vi "SOAE-Initialize Hardware.vi"(0 "Params":T1, 11 "error in (no error)":errorcluster) -> (4 "task out":refnum<k21>, 15 "error out":errorcluster)   [LabVIEW 2020]
uses:
  Typedefs/SOAE-Parameters.ctl
  Misc VIs/Connection Manager/Type Defs/Input sources.ctl
  <vilib>/DAQmx/create/channels.llb/DAQmx Create Channel (AI-Voltage-Basic).vi
  <vilib>/DAQmx/configure/timing.llb/DAQmx Timing (Sample Clock).vi
  <resource>/objmgr/daqmx.rc
panel:
  in  "input terminal configuration":i32(ring)=-1 items=["Default"=-1, "RSE"=10083, "NRSE"=10078, "Differential"=10106, "Pseudodifferential"=12529]
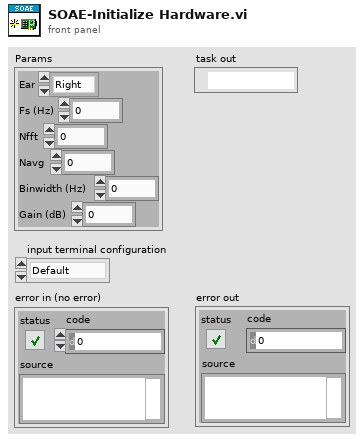
[diagram p1: front panel]
types:
  T1 = typedef "SOAE-Parameters.ctl" = cluster{"Ear":enum16{"Right", "Left"}, "Fs (Hz)":dbl, "Nfft":i32, "Navg":i32, "Binwidth (Hz)":dbl, "Gain (dB)":dbl}
  T2 = typedef "Input sources.ctl" = u16
  T3 = typedef "PXI-Device Spec.ctl" = cluster{"Slot":i32, "ProductType":string, "NumAO":i32, "NumAI":i32, "Device Name":string}
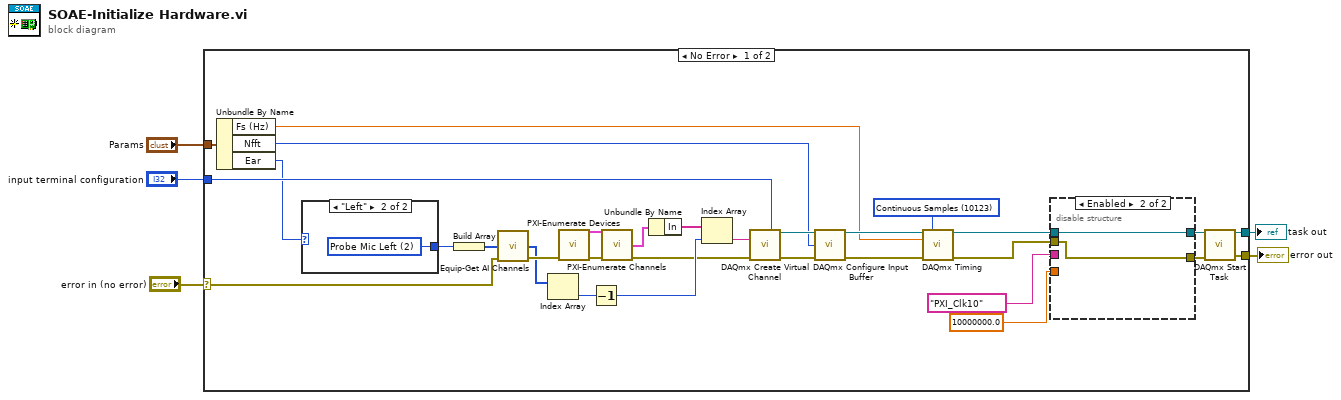
[diagram p0: block diagram]
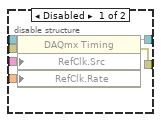
[diagram p2: hidden frame]
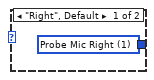
[diagram p3: hidden frame]
diagram:
  n1 = case shown="No Error" "error in (no error)" {
    selector: "error in (no error)" -> [w6 w47]
    tunnel: "input terminal configuration" -> [w36 _]
    tunnel: [w31 _] -> w4
    tunnel: [w23 w47] -> w3
    tunnel: "Params" -> [w22 _]
    frame No Error {
      w30 = 10123 items=["Finite Samples"=10178, "Continuous Samples"=10123, "Hardware Timed Single Point"=12522] ("sample mode")
      n2 = Unbundle By Name(w22) -> ("Fs (Hz)"=w21:dbl, "Nfft"=w20:i32, "Ear"=w17:enum16{"Right", "Left"})
      n3 = case shown="\"Left\"" w17 {
        tunnel: [w45 w46] -> w16
        frame "Right", Default {
          w45 = T2 1 items=["--unused--", "Probe Mic Right", "Probe Mic Left", "Cal Mic", "ABR", "CAP Right", "CAP Left", "Startle piezo", "Temperature", "Heart rate", "Accelerometer"] ("Ring")
        }
        frame "Left" {
          w46 = T2 2 items=["--unused--", "Probe Mic Right", "Probe Mic Left", "Cal Mic", "ABR", "CAP Right", "CAP Left", "Startle piezo", "Temperature", "Heart rate", "Accelerometer"] ("Ring")
        }
      }
      n4 = Build Array(w16) -> (w15:T2[])
      n5 = call "Equip-Get AI Channels.vi"("Inputs"=w15, "error in (no error)"=w6) -> ("AI Channels"=w11:i32[], "error out"=w14:errorcluster)  [unwired: 12 in]
      n6 = Index Array(array=w11) -> (element=w10:i32)  [unwired: 1 in]
      n7 = call "PXI-Enumerate Devices.vi"("error in (no error)"=w14) -> ("Devices"=w18:T3[], "error out"=w19:errorcluster)  [unwired: 13 in]
      n8 = Decrement(x=w10) -> (x-1=w9:i32)
      n9 = call "PXI-Enumerate Channels.vi"("Devices"=w18, "error in (no error)"=w19) -> ("Channels (1D)"=w13:cluster{"Out":string[], "In":string[]}, "error out"=w8:errorcluster)  [unwired: 11 in, 1 out]
      n10 = Unbundle By Name(w13) -> ("In"=w12:string[])
      n11 = Index Array(array=w12, index=w9) -> (element=w7:string)
      n12 = call-poly <vilib>:"DAQmx Create Virtual Channel.vi"("input terminal configuration"=w36, "physical channels"=w7, "error in"=w8) -> ("task out"=w32:refnum<k21>, "error out"=w33:errorcluster)  [unwired: 11 in]
      n13 = call <vilib>:"DAQmx Configure Input Buffer.vi"("task/channels in"=w32, "buffer size (in samples per channel)"=w20, "error in"=w33) -> ("task out"=w34:refnum<k21>, "error out"=w35:errorcluster)  [unwired: 11 in]
      n14 = call-poly <vilib>:"DAQmx Timing.vi"("task/channels in"=w34, "sample mode"=w30, "rate"=w21, "error in"=w35) -> ("task out"=w27:refnum<k21>, "error out"=w25:errorcluster)  [unwired: 10 in]
      n15 = disable-structure shown="Enabled" {
        disable-tunnel: 10000000.0 -> [w42 _]
        disable-tunnel: tag "PXI_Clk10" ("RefClk.Src") -> [w41 _]
        disable-tunnel: w27 -> [w40 w44]
        disable-tunnel: [w39 w44] -> w26
        disable-tunnel: w25 -> [w38 w43]
        disable-tunnel: [w37 w43] -> w24
        frame Disabled {
          n16 = property class="DAQmx Timing"(reference=w40, error in=w38, "RefClk.Src"=w41, "RefClk.Rate"=w42) -> (reference out=w39:refnum<k21>, error out=w37:errorcluster)
        }
        frame Enabled {
        }
      }
      n17 = call <vilib>:"DAQmx Start Task.vi"("task/channels in"=w26, "error in"=w24) -> ("task out"=w31:refnum<k21>, "error out"=w23:errorcluster)  [unwired: 12 in]
    }
    frame Error {
    }
  }
  "error out" <- w3
  "task out" <- w4
